vi "Main Dialog.vi"() -> ()   [LabVIEW 2020, in "Process Generation.lvlib" / "New Class Dialog.lvclass"]
uses:
  New Class Dialog.lvclass
  Tag Tree Helper/Tag Tree Helper.lvclass
  Tag Tree Helper/Tag Tree Helper.lvclass/Tag Tree Helper.ctl
  New Class Dialog.lvclass/New Class Dialog.ctl
  Process Generator/Process Generator.lvclass/Process Generator.ctl
  Process Generator/Private/Generate Random Material Design Color.vi
  Process Generator/Process Generator.lvclass
panel:
  in  "Parent Class":string(tree)
  in  "Process Name":string
  in  "Save to Folder":path
  in  "Commit":bool
  in  "Cancel":bool
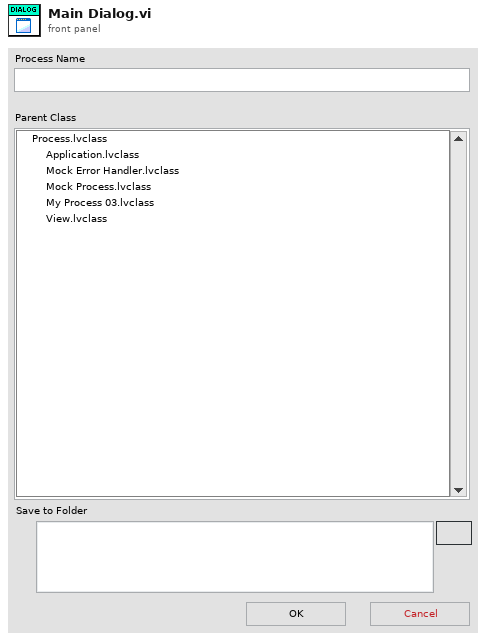
[diagram p1: front panel]
types:
  T1 = enum8{"Enabled", "Disabled", "Disabled and Grayed Out"}
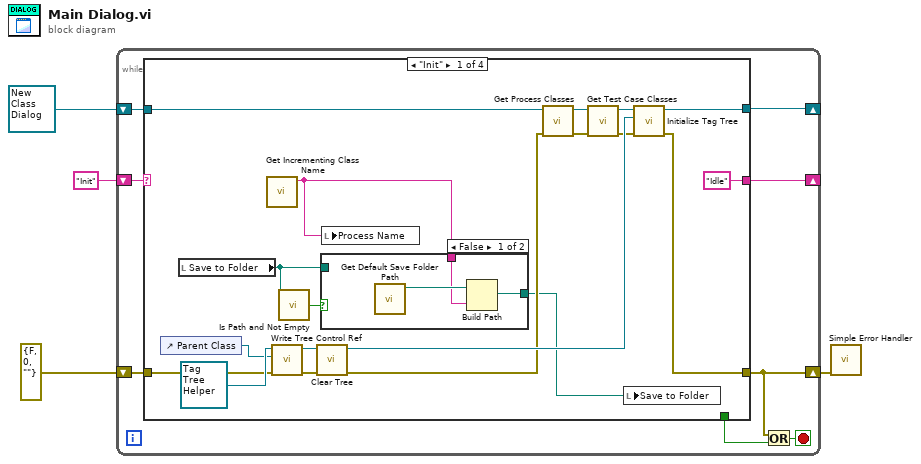
[diagram p0: block diagram]
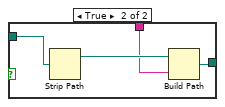
[diagram p2: hidden frame]
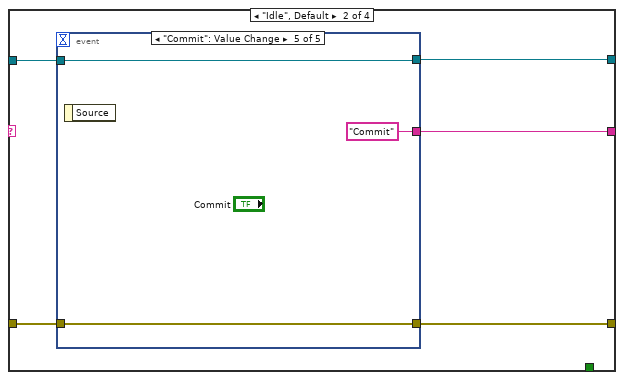
[diagram p3: hidden frame]
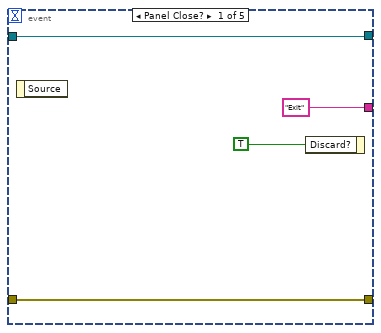
[diagram p4: hidden frame]
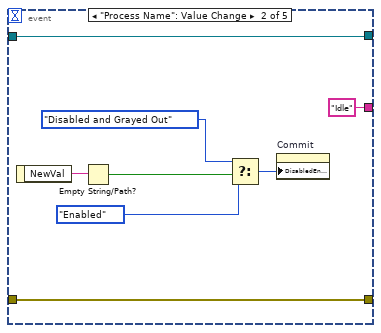
[diagram p5: hidden frame]
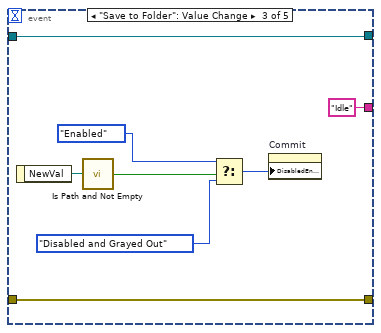
[diagram p6: hidden frame]
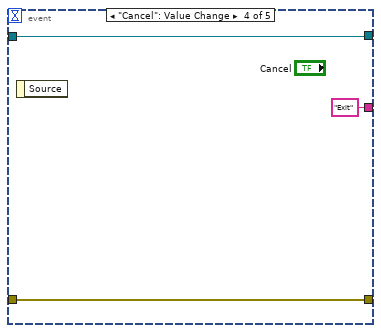
[diagram p7: hidden frame]
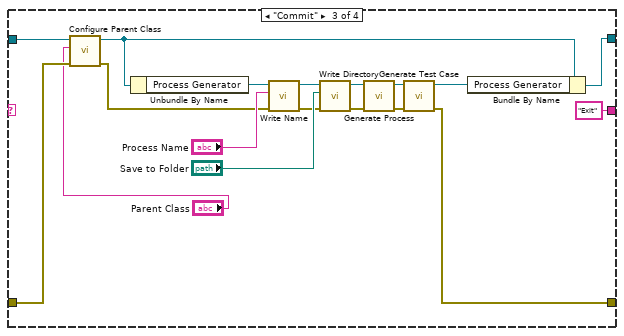
[diagram p8: hidden frame]
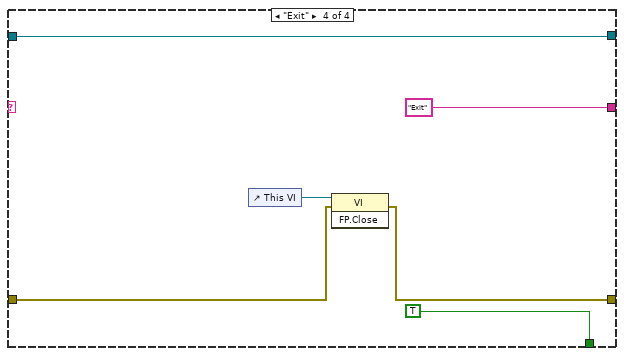
[diagram p9: hidden frame]
diagram:
  n1 = while {
    shift-right: [w9] -> _
    shift-left: refnum<class "New Class Dialog.lvclass"> refnum ("New Class Dialog In") -> [w10]
    shift-right: [w5] -> w2
    shift-left: errorcluster {"status"=FALSE, "code"=0, "source"=""} ("error in (no error)") -> [w11]
    shift-right: [w8] -> _
    shift-left: "Init" -> [w12]
    stop <- w6 stop-if-true
    n2 = case shown="\"Init\"" w12 {
      tunnel: [w25 w43 w74 w89] -> w5
      tunnel: w11 -> [w22 w42 w76 w88]
      tunnel: w10 -> [w30 w41 w72 w93]
      tunnel: [w27 w40 w75 w93] -> w9
      tunnel: ["Idle" w39 "Exit" "Exit"] -> w8
      tunnel: [_ _ _ TRUE] -> w7
      frame "Init" {
        n3 = control-ref of="Parent Class"() -> (w28:refnum<vi>)
        n4 = local read "Save to Folder"() -> (w20:path)
        n5 = call "Get Incrementing Class Name.vi"() -> ("String"=w19:string)  [unwired: 11 in]
        n6 = call "Write Tree Control Ref.vi"("error in (no error)"=w22, "Tag Tree Reference"=w28, "Tag Tree Helper In"=refnum<class "Tag Tree Helper.lvclass"> refnum ("Support Utilities.lvlib:Tag Tree.lvclass")) -> ("error out"=w26:errorcluster, "Tag Tree Helper Out"=w23:refnum<class "Tag Tree Helper.lvclass">)  [unwired: 7 in]
        n7 = call <vilib>:"Is Path and Not Empty.vi"("path"=w20) -> ("Is Path and Not Empty?"=w18:bool)  [unwired: 4 in]
        n8 = call "Clear Tree.vi"("error in (no error)"=w26, "Tag Tree Helper In"=w23) -> ("error out"=w21:errorcluster, "Tag Tree Helper Out"=w24:refnum<class "Tag Tree Helper.lvclass">)  [unwired: 8 in]
        n9 = case shown="False" w18 {
          tunnel: w20 -> [_ w38]
          tunnel: w19 -> [w33 w36]
          tunnel: [w32 w35] -> w17
          frame False {
            n10 = call "Get Default Save Folder Path.vi"() -> ("Path"=w34:path)  [unwired: 11 in]
            n11 = Build Path(base path=w34, name or relative path=w33) -> (appended path=w32:path)
          }
          frame True {
            n12 = Strip Path(path=w38) -> (stripped path=w37:path)  [unwired: 1 out]
            n13 = Build Path(base path=w37, name or relative path=w36) -> (appended path=w35:path)
          }
        }
        n14 = local write "Process Name"(w19) -> ()
        n15 = call "Get Process Classes.vi"("error in (no error)"=w21, "New Class Dialog In"=w30) -> ("error out"=w15:errorcluster, "New Class Dialog Out"=w16:refnum<class "New Class Dialog.lvclass">)  [unwired: 8 in]
        n16 = call "Get Test Case Classes.vi"("error in (no error)"=w15, "New Class Dialog In"=w16) -> ("error out"=w13:errorcluster, "New Class Dialog Out"=w14:refnum<class "New Class Dialog.lvclass">)  [unwired: 8 in]
        n17 = local write "Save to Folder"(w17) -> ()
        n18 = call "Initialize Tag Tree.vi"("error in (no error)"=w13, "Tag Tree Helper"=w24, "New Class Dialog In"=w14) -> ("error out"=w25:errorcluster, "New Class Dialog Out"=w27:refnum<class "New Class Dialog.lvclass">)  [unwired: 7 in]
      }
      frame "Idle", Default {
        n19 = event shown="[4] \"Commit\": Value Change" {
          selector: _ -> [_ _ _ _ _]
          dyn-events: _ -> [_ _ _ _ _]
          timeout: _ -> [_ _ _ _ _]
          tunnel: [w47 w55 w63 w65 w69] -> w43
          tunnel: w42 -> [w47 w55 w63 w65 w69]
          tunnel: w41 -> [w46 w54 w62 w66 w68]
          tunnel: [w46 w54 w62 w66 w68] -> w40
          tunnel: ["Exit" "Idle" "Idle" "Exit" "Commit"] -> w39
          event Panel Close? {
            n20 = event-data() -> ()  [unwired: 1 in, 1 out]
            n21 = event-data("Discard?"=TRUE) -> ()  [unwired: 1 in, 1 out]
          }
          event "Process Name": Value Change {
            n22 = event-data() -> ("NewVal"=w53:string)  [unwired: 1 in]
            n23 = Empty String/Path?(string/path=w53) -> (empty?=w52:bool)
            n24 = Select(t=T1."Disabled and Grayed Out" ("Disabled"), s=w52, f=T1."Enabled") -> (s? t:f=w49:T1)
            n25 = property on="Commit" class="Bool"("DisabledEnum"=w49) -> ()  [unwired: 2 in, 2 out]
          }
          event "Save to Folder": Value Change {
            n26 = event-data() -> ("NewVal"=w61:path)  [unwired: 1 in]
            n27 = call <vilib>:"Is Path and Not Empty.vi"("path"=w61) -> ("Is Path and Not Empty?"=w60:bool)  [unwired: 4 in]
            n28 = Select(t=T1."Enabled" ("f"), s=w60, f=T1."Disabled and Grayed Out" ("Disabled")) -> (s? t:f=w57:T1)
            n29 = property on="Commit" class="Bool"("DisabledEnum"=w57) -> ()  [unwired: 2 in, 2 out]
          }
          event "Cancel": Value Change {
            n30 = event-data() -> ()  [unwired: 1 in, 1 out]
          }
          event "Commit": Value Change {
            n31 = event-data() -> ()  [unwired: 1 in, 1 out]
          }
        }
      }
      frame "Commit" {
        n32 = call "Configure Parent Class.vi"("error in (no error)"=w76, "Parent Class"="Parent Class", "New Class Dialog In"=w72) -> ("error out"=w73:errorcluster, "New Class Dialog Out"=w71:refnum<class "New Class Dialog.lvclass">)  [unwired: 7 in]
        n33 = Unbundle By Name(w71) -> ("Process Generator"=w84:refnum<class "Process Generator.lvclass">)
        n34 = call "Write Name.vi"("error in (no error)"=w73, "Name"="Process Name", "Process Generator In"=w84) -> ("error out"=w82:errorcluster, "Process Generator Out"=w83:refnum<class "Process Generator.lvclass">)  [unwired: 7 in]
        n35 = call "Write Directory.vi"("error in (no error)"=w82, "Directory"="Save to Folder", "Process Generator in"=w83) -> ("error out"=w80:errorcluster, "Process Generator out"=w81:refnum<class "Process Generator.lvclass">)  [unwired: 7 in]
        n36 = call "Generate Process.vi"("error in (no error)"=w80, "Process Generator In"=w81) -> ("error out"=w78:errorcluster, "Process Generator Out"=w79:refnum<class "Process Generator.lvclass">)  [unwired: 8 in]
        n37 = call "Generate Test Case.vi"("error in (no error)"=w78, "Process Generator In"=w79) -> ("error out"=w74:errorcluster, "Process Generator Out"=w77:refnum<class "Process Generator.lvclass">)  [unwired: 8 in]
        n38 = Bundle By Name(cluster=w71, "Process Generator"=w77) -> (w75:refnum<class "New Class Dialog.lvclass">)
      }
      frame "Exit" {
        n39 = control-ref of="This VI"() -> (w90:refnum<vi>)
        n40 = invoke class="VI" method="FP.Close"(reference=w90, error in=w88) -> (error out=w89:errorcluster)  [unwired: 1 in, 2 out]
      }
    }
    n41 = Or(x=w5, y=w7) -> (x .or. y?=w6:bool)
  }
  n42 = call <vilib>:"Simple Error Handler.vi"("error in (no error)"=w2) -> ()  [unwired: 4 in, 5 out]
